vi "9 - Workbook from template.vi"() -> ()   [LabVIEW 2020]
uses:
  client/client.lvlib
panel:
  out "workbook names":string[](array[string])
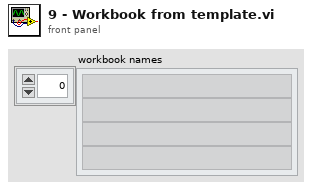
[diagram p1: front panel]
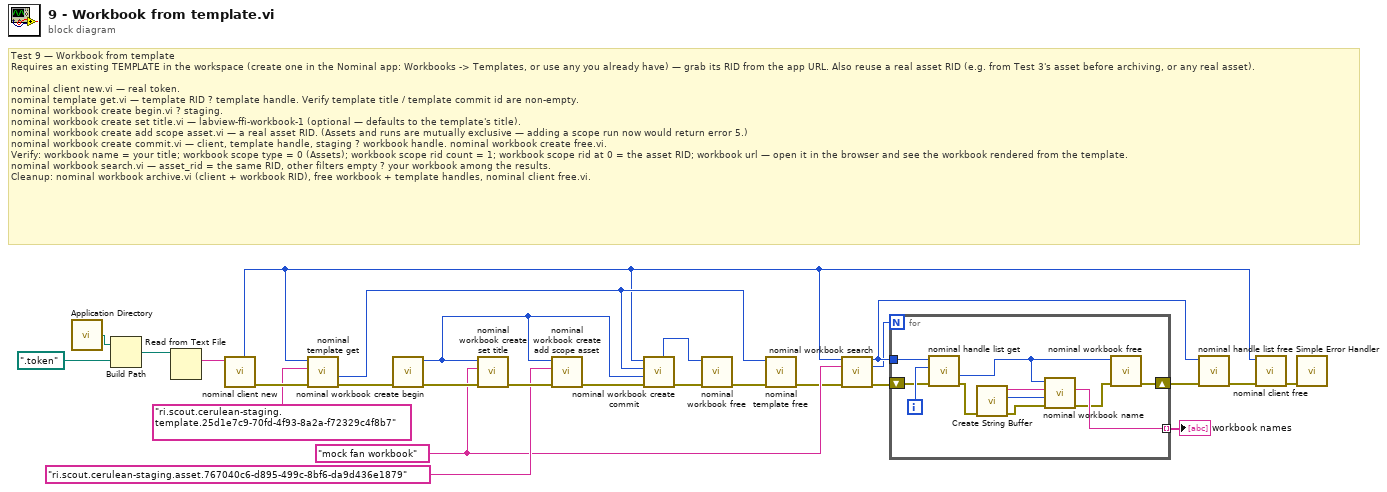
[diagram p0: block diagram]
diagram:
  w9 = "mock fan workbook" ("title")
  # "Test 9 — Workbook from template\nRequires an existing TEMPLATE in the workspace (create one in the Nominal app: Workbooks -> Templates, or use any you already have) — grab its RID from the app URL. Also reuse a real asset RID (e.g. from Test 3's asset before archiving, or any real asset).\n\nnominal client new.vi — real token.\nnominal template get.vi — template RID ? template handle. Verify template title / template commit id are non-empty.\nnominal workbook create begin.vi ? staging.\nnominal workbook create set title.vi — labview-ffi-workbook-1 (optional — defaults to the template's title).\nnominal workbook create add scope asset.vi — a real asset RID. (Assets and runs are mutually exclusive — adding a scope run now would return error 5.)\nnominal workbook create commit.vi — client, template handle, staging ? workbook handle. nominal workbook create free.vi.\nVerify: workbook name = your title; workbook scope type = 0 (Assets); workbook scope rid count = 1; workbook scope rid at 0 = the asset RID; workbook url — open it in the browser and see the workbook rendered from the template.\nnominal workbook search.vi — asset_rid = the same RID, other filters empty ? your workbook among the results.\nCleanup: nominal workbook archive.vi (client + workbook RID), free workbook + template handles, nominal client free.vi."
  n1 = call <vilib>:"Application Directory.vi"() -> ("Application Directory"=w26:path)
  n2 = Build Path(base path=w26, name or relative path=path ".token") -> (appended path=w24:path)
  n3 = Read from Text File(file (use dialog)=w24) -> (text=w23:string)  [unwired: 3 in, 3 out]
  n4 = call "nominal client new.vi"("token"=w23) -> ("error out"=w21:errorcluster, "out_client out"=w8:i32)  [unwired: 8 in, 1 out]
  n5 = call "nominal template get.vi"("error in (no error)"=w21, "rid"="ri.scout.cerulean-staging.template.25d1e7c9-70fd-4f93-8a2a-f72329c4f8b7", "client"=w8) -> ("error out"=w20:errorcluster, "out_template out"=w15:i32)  [unwired: 6 in, 1 out]
  n6 = call "nominal workbook create begin.vi"("error in (no error)"=w20) -> ("error out"=w19:errorcluster, "out_staging out"=w16:i32)  [unwired: 8 in, 1 out]
  n7 = call "nominal workbook create set title.vi"("error in (no error)"=w19, "title"=w9, "staging"=w16) -> ("error out"=w18:errorcluster)  [unwired: 7 in, 1 out]
  n8 = call "nominal workbook create add scope asset.vi"("error in (no error)"=w18, "asset_rid"="ri.scout.cerulean-staging.asset.767040c6-d895-499c-8bf6-da9d436e1879" ("title"), "staging"=w16) -> ("error out"=w17:errorcluster)  [unwired: 7 in, 1 out]
  n9 = call "nominal workbook create commit.vi"("error in (no error)"=w17, "staging"=w16, "template_"=w15, "client"=w8) -> ("error out"=w12:errorcluster, "out_workbook out"=w14:i32)  [unwired: 5 in, 1 out]
  n10 = call "nominal workbook free.vi"("error in (no error)"=w12, "workbook"=w14) -> ("error out"=w13:errorcluster)  [unwired: 8 in, 1 out]
  n11 = call "nominal template free.vi"("error in (no error)"=w13, "template_"=w15) -> ("error out"=w7:errorcluster)  [unwired: 8 in, 1 out]
  n12 = call "nominal workbook search.vi"("client"=w8, "search_text"=w9, "error in (no error)"=w7) -> ("out_list out"=w5:i32, "out_count out"=w2:u32, "error out"=w6:errorcluster)  [unwired: 9 in, 1 out]
  n13 = for {
    N: w2 -> [_]
    tunnel: w5 -> [w37]
    shift-right: [w33] -> w4
    shift-left: w6 -> [w35]
    tunnel: [w28] -> w1 mode=indexing
    i -> [w36]
    n14 = call "nominal handle list get.vi"("error in (no error)"=w35, "index"=w36, "list"=w37) -> ("error out"=w34:errorcluster, "out_handle out"=w32:i32)  [unwired: 6 in, 1 out]
    n15 = call "Create String Buffer.vi"("error in"=w34) -> ("error out"=w29:errorcluster, "dub Buffer Size"=w30:i32, "String Buffer"=w31:string)  [unwired: 8 in]
    n16 = call "nominal workbook name.vi"("error in (no error)"=w29, "cap"=w30, "buf"=w31, "workbook"=w32) -> ("error out"=w27:errorcluster, "buf out"=w28:string)  [unwired: 4 in, 2 out]
    n17 = call "nominal workbook free.vi"("error in (no error)"=w27, "workbook"=w32) -> ("error out"=w33:errorcluster)  [unwired: 8 in, 1 out]
  }
  "workbook names" <- w1
  n18 = call "nominal handle list free.vi"("error in (no error)"=w4, "list"=w5) -> ("error out"=w3:errorcluster)  [unwired: 8 in, 1 out]
  n19 = call "nominal client free.vi"("error in (no error)"=w3, "client"=w8) -> ("error out"=w22:errorcluster)  [unwired: 8 in, 1 out]
  n20 = call <vilib>:"Simple Error Handler.vi"("error in (no error)"=w22) -> ()  [unwired: 4 in, 5 out]
